vi "extract.vi"   [LabVIEW 2015, in "lv-bin-7zip.lvlib" / "v1.lvlib"]
doc: "this can be used to extract one or more files from an archive, it also has the ability to \"preview\" files that would be extracted from an archive rather than actually extract them."
uses:
  v1.lvlib
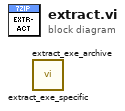
[diagram p0: block diagram]
diagram:
  n1 = call "extract_exe_specific.vi"() -> ()  [unwired: 9 in, 3 out]
  n2 = call "extract_exe_archive.vi"() -> ()  [unwired: 8 in, 4 out]
